vi "FPGA_OffResonanceTapping-SlowScanner.vi"() -> ()   [LabVIEW 2016]
uses:
  <vilib>/rvi/DataTransferAndStorage/Container/XNode/niFpgaContainer.xnode
  <vilib>/rvi/Memory/Memory_Emulation/nirvimemoryEmulation.vi
  <vilib>/rvi/Memory/Memory_Emulation/nirvimemoryFastEmulation.vi
  <vilib>/Platform/TimedLoop/XDataNode/wakeup.ctl
  <vilib>/Platform/TimedLoop/XDataNode/XDNodeRunTimeDep.lvlib
  <vilib>/Platform/TimedLoop/XDataNode/nitl_modes.ctl
  <vilib>/Platform/TimedLoop/XDataNode/timing_clust.ctl
  <vilib>/Platform/TimedLoop/XDataNode/XDataNode.xnode
  <vilib>/eio/EIONode/EIONode.xnode
  <vilib>/rvi/eio/common/nirviEmuTemplateMethod_errors.vi
  <vilib>/rvi/DataTransferAndStorage/Handshake/Emulation/niFpgaHandshakeEmulation.vi
  <vilib>/rvi/FIFO/Fifo_Resource/nirvififoEmulationWrite.vi
  <vilib>/rvi/FIFO/Fifo_Resource/nirvififoEmulationRead.vi
  <vilib>/rvi/FXPMathLib/FxpAdd/XNode/nifxpmath_Add.xnode
  <vilib>/rvi/FXPMathLib/sim/FxpSim.dll
  <instrlib>/_niInstr/Basic Elements/v1/FPGA/niInstr Basic Elements v1 FPGA.lvlib
  <vilib>/rvi/DataTransferAndStorage/Register/Emulation/niFpgaRegisterEmulation.vi
  <vilib>/rvi/interface/RandomDataEmulation/nirviRandomDataFpgaReadWriteTemplate.vi
  <vilib>/rvi/FXPMathLib/FxpInterpret/XNode/nifxpmath_Interpret.xnode
  <vilib>/rvi/FXPMathLib/FxpSub/XNode/nifxpmath_Sub.xnode
  <vilib>/rvi/FXPMathLib/FxpMul/XNode/nifxpmath_Multiplier.xnode
panel:
  out "ticksPerPixel 2":u32
  in  "Tab Control":T1(tab)
  in  "fastBlanking":T2={"startFwd"=0, "endFwd"=10000, "startBwd"=0, "endBwd"=0, "disableBlanking"=FALSE}
  in  "scanRates":T3={"outputRate"=50, "fastDecFactor"=0, "outWaveSizeFast"=0, "pplUpsampling"=0, "numLines"=0}
  in  "scanSize":T4
  in  "outputMatrix":T5
  in  "singleDirectionScan":bool
  in  "scanOffset":cluster{"x":fxp<+/-,16,1>, "y":fxp<+/-,16,1>}
  in  "scanEnabled":bool
  out "actualOutputRate":u32
  in  "fastDecFactorInv":fxp<+,22,0>
  in  "slowUpStep":fxp<+,22,0>
  in  "outWaveSizeSlow":u16
  in  "moveRates":T6
  out "isSlowlyMoving?":bool
  in  "invMoveToDec":fxp<+,16,0>
  in  "moveToPoint":cluster{"x":fxp<+/-,16,1>, "y":fxp<+/-,16,1>}
  in  "doSlowMove":bool
  in  "enableFeedback":bool
  out "zHeightFlt":fxp<+/-,20,2>
  in  "feedbackParams":T7={"setPoint"=0.001007080078125, "pGain"=0.0, "iGain"=0.10000038146972656, "gainScale"=3}
  in  "liftOffParams":T8={"liftHeight"=0.0498046875, "disengagePos"=-1.0}
  out "isPIDatLimit?":bool
  out "inputPID":fxp<+/-,24,1> format="%#_6p"
  out "inputPIDnoRescale":fxp<+/-,24,16>
  in  "manualMotionZ":T9
  out "isManualPIDMoving?":bool
  out "zHeight":fxp<+/-,28,1>
  in  "limits":T10={"upperLimit"=2.0, "lowerLimit"=0.0}
  in  "stepMot.HalfStep":T11={"Address (0-7)"=0, "stateData"=[TRUE, FALSE, FALSE, FALSE], "isWritingToMotor?"=FALSE}
  in  "stepMot.Address(0-7)":i8
  in  "scannerTimeConstant":u32=1000 caption="scanner Time Constant [us]"
  in  "resetBGC":bool
  in  "bgSatCntP2":u16=12
  in  "bgcWaitTicks":u32
  in  "allowPXIBGC":bool
  out "output":cluster{"index":u16, "data":i16}
  out "interactionMaxOut":fxp<+/-,24,16>
  in  "waveLength":u16=5000
  out "readInteraction":i16
  out "readBackground":i16
  in  "readBackgroundAddress":u32
  in  "Count(mSec)":u32=200 caption="updateRateMs"
  in  "intOutMAEnable":bool
  in  "intOutMAExpFactor":i8=-4
  in  "fittingParams":T12={"maxLoc"=0, "threshold"=0, "fitHardPtLimit"=5000}
  in  "outWaveWrite":cluster{"write":bool, "data":i16, "index":u16}
  in  "fitWeightsWrite":T13
  in  "fitFactorWrite":T14
  in  "moveWaveWrite":T15
  in  "moveToWaveWrite":T16
  in  "slowWaveWrite":T17
  in  "fastWaveWrite":T17
  out "X (fast)":i16
  out "Y (slow)":i16
  in  "sosBypass":bool[](array[boolean])=[FALSE, FALSE, FALSE, FALSE, FALSE, FALSE, FALSE, FALSE]
  in  "anot":fxp<+/-,24,5>[](array[numeric])=[0.0, 0.0, 0.0, 0.0, 0.0, 0.0, 0.0, 0.0, 0.0, 0.0, 0.0, 0.0, 0.0, 0.0, 0.0, 0.0]
  in  "b":fxp<+/-,24,5>[](array[numeric])=[0.0, 0.0, 0.0, 0.0, 0.0, 0.0, 0.0, 0.0, 0.0, 0.0, 0.0, 0.0, 0.0, 0.0, 0.0, 0.0, 0.0, 0.0, 0.0, 0.0, 0.0, 0.0, 0.0, 0.0]
  in  "enableOutputSS":bool
  in  "outputSSRate":u16=1000
  out "ticksPerPixel":u32
  out "hostTransferOverflow":bool
  in  "transferInteraction":bool
  in  "syncDecimation":u16=50
  in  "zeroInput":bool
  in  "bypassMaxAveraging":bool
  out "savedPoint":T18
  in  "EnableExcitation":bool
  in  "piezoMode":bool
  in  "invertOutput":bool
  in  "invertInput":bool
  in  "maxSearchBounds":T19={"maxSearchLower"=200, "maxSearchUpper"=600}
  in  "useSyncPoint":bool
  in  "syncPoint":u16
  in  "syncAverageBand":u16=2 caption="syncAverageBand (2^n)"
  out "maxSearchIndex":u16
  in  "zDataRate":u32=45 caption="Count(Ticks)"
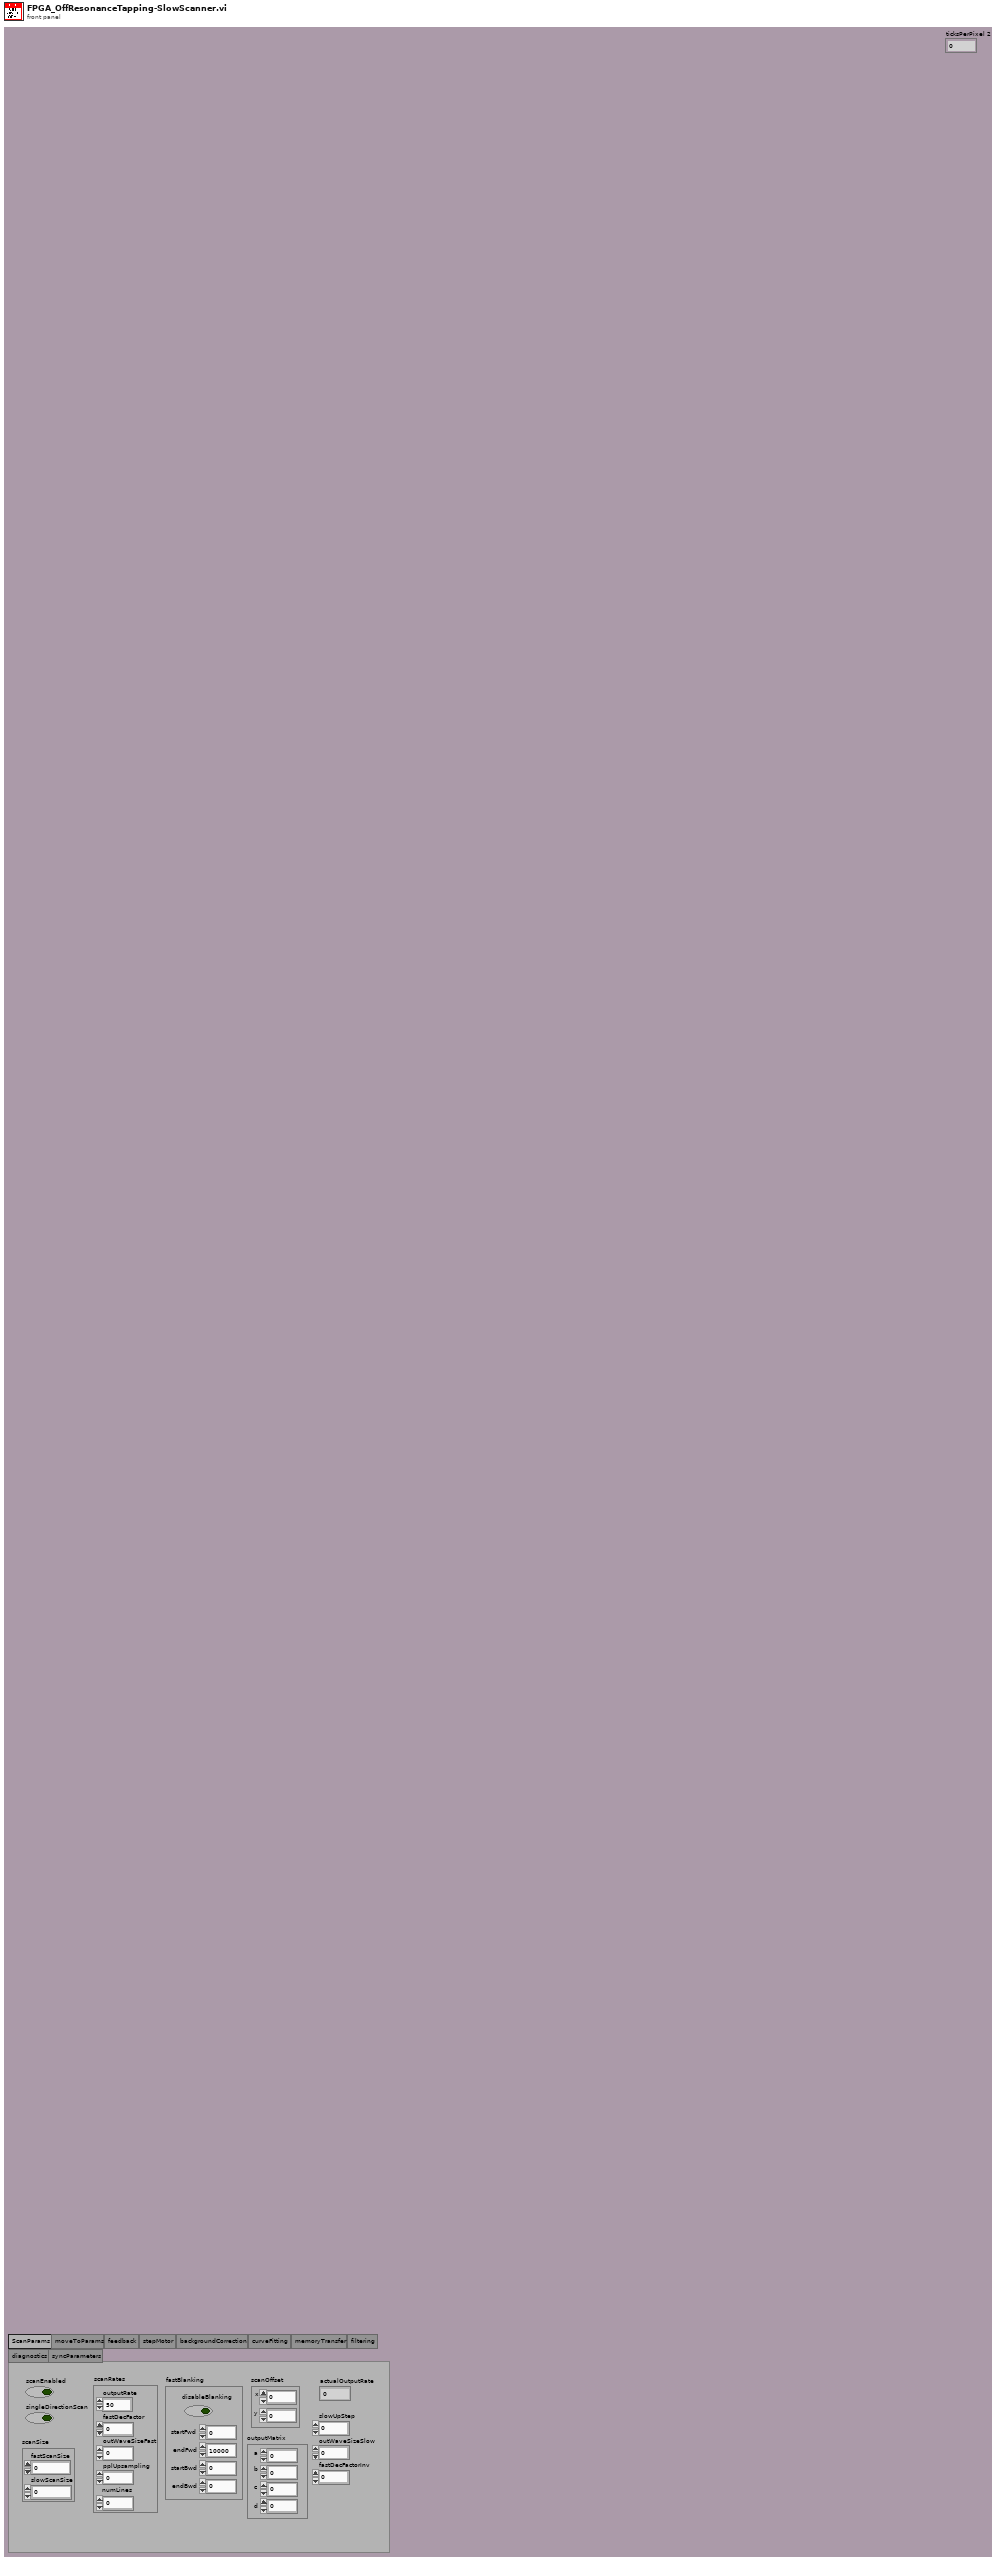
[diagram p1: front panel]
types:
  T1 = enum32{"ScanParams", "moveToParams", "feedback", "stepMotor", "backgroundCorrection", "curveFitting", "memoryTransfer", "filtering", "diagnostics", "syncParameters"}
  T2 = cluster{"startFwd":u16, "endFwd":u16, "startBwd":u16, "endBwd":u16, "disableBlanking":bool}
  T3 = cluster{"outputRate":u16, "fastDecFactor":u16, "outWaveSizeFast":u16, "pplUpsampling":u16, "numLines":u16}
  T4 = cluster{"fastScanSize":fxp<+,17,1>, "slowScanSize":fxp<+,17,1>}
  T5 = cluster{"a":fxp<+/-,18,2>, "b":fxp<+/-,18,2>, "c":fxp<+/-,18,2>, "d":fxp<+/-,18,2>}
  T6 = cluster{"moveToDecFactor":u16, "moveToWaveSize":u16}
  T7 = cluster{"setPoint":fxp<+/-,17,1>, "pGain":fxp<+/-,20,1>, "iGain":fxp<+/-,20,1>, "gainScale":i8}
  T8 = cluster{"liftHeight":fxp<+/-,15,4>, "disengagePos":fxp<+/-,22,1>}
  T9 = cluster{"enableManualMotion":bool, "doMove":bool, "integratorTarget":fxp<+/-,22,2>, "moveDecimation":u16, "moveWaveSize":u16}
  T10 = cluster{"upperLimit":fxp<+/-,28,4>, "lowerLimit":fxp<+/-,28,4>}
  T11 = cluster{"Address (0-7)":u8, "stateData":bool[], "isWritingToMotor?":bool}
  T12 = cluster{"maxLoc":u16, "threshold":i16, "fitHardPtLimit":u16}
  T13 = cluster{"write":bool, "data":fxp<+,20,0>, "index":u16}
  T14 = cluster{"write":bool, "index":u16, "fitCoefficients":cluster{"a":fxp<+/-,21,7>, "b":fxp<+/-,21,7>, "factorA":i8, "factorB":i8}}
  T15 = cluster{"write":bool, "data":fxp<+,16,1>, "index":u16}
  T16 = cluster{"write":bool, "index":u16, "data":fxp<+/-,18,1>}
  T17 = cluster{"write":bool, "index":u16, "data":fxp<+/-,18,2>}
  T18 = cluster{"xOut":fxp<+/-,18,2>, "yOut":fxp<+/-,18,2>}
  T19 = cluster{"maxSearchLower":u16, "maxSearchUpper":u16}
  T20 = typedef "XDNodeRunTimeDep.lvlib/timing_clust.ctl" = cluster{"Expected End [f-1]":u64, "Actual End [f-1]":u64, "Finished Late? [f-1]":bool, "Expected End [i-1]":u64, "Actual End [i-1]":u64, "Finished Late? [i-1]":bool, "Expected Start [i]":u64, "Actual Start [i]":u64, "Expected Start [f]":u64, "Actual Start [f]":u64, "Source Name":string, "Structure Name":string, "Period":i64, "Deadline":i64, "Offset":i64, "Start":i64, "Priority":i32, "Timeout":i32, "Mode":T21, "Wakeup Reason":T22, "Error":errorcluster, "Source Type":string, "Secondary Source Type":string, "Global End Time":u64, "Global Start Time":u64, "Frame Duration":u64, "Iteration Duration":u64, "Assigned CPU":i32, "I/O Scan Engine Mode":u32}
  T21 = typedef "XDNodeRunTimeDep.lvlib/nitl_modes.ctl" = enum32{"No Change", "Process missed periods, maintain original phase", "Discard missed periods, maintain original phase", "Process missed periods, ignore original phase", "Discard missed periods, ignore original phase"}
  T22 = typedef "XDNodeRunTimeDep.lvlib/wakeup.ctl" = enum32{"Normal", "Aborted", "Asynchronous wakeup", "Timing source error", "Timed loop error", "Timeout"}
  T23 = cluster{"linSum":i32, "wtSum":fxp<+/-,54,34>, "count":u16, "forward":bool}
  T24 = cluster{cluster{"outMinFwd":fxp<+,22,1>, "outMinBwd":fxp<+,22,1>}, "outputValid":bool}
  T25 = cluster{"Element":cluster{"a":i32, "b":i32}, "outputValid":bool}
  T26 = cluster{"Element":cluster{"linSum":i32, "wtSum":fxp<+/-,54,34>, "count":u16}, "outputValid":bool}
  T27 = cluster{"outMinFwd":fxp<+,22,1>, "outMinBwd":fxp<+,22,1>}
  T28 = cluster{"linSum":i32, "wtSum":fxp<+/-,54,34>, "count":u16}
  T29 = cluster{"enable":bool, "setPoint":fxp<+/-,17,1>, "pGain":fxp<+/-,20,1>, "iGain":fxp<+/-,20,1>, "gainScale":i8}
  T30 = cluster{"liftHeight":fxp<+/-,15,4>, "disengagePos":fxp<+/-,22,1>, "liftOff":bool}
  T31 = cluster{"zHeight":fxp<+/-,28,1>, "integer_zHeight":i16, "error":fxp<+/-,25,2>, "pidAtLimit":bool, "moving":bool}
  T32 = cluster{"a":fxp<+/-,21,7>, "b":fxp<+/-,21,7>, "factorA":i8, "factorB":i8}
  T33 = cluster{"output":bool, "fastIndex":bool, "line":bool, "frame":bool, "moveIndex":bool, "moveDone":bool, "pixel":bool}
  T34 = cluster{"interpOutput":fxp<+/-,19,2>, "interpOutput":fxp<+/-,19,2>}
  T35 = cluster{"x+y":fxp<+/-,18,2>, "x+y":fxp<+/-,18,2>}
  T36 = cluster{"[0]":bool, "[1]":bool, "[2]":bool, "[3]":bool, "[4]":bool, "[5]":bool, "[6]":bool, "[7]":bool, "[8]":bool}
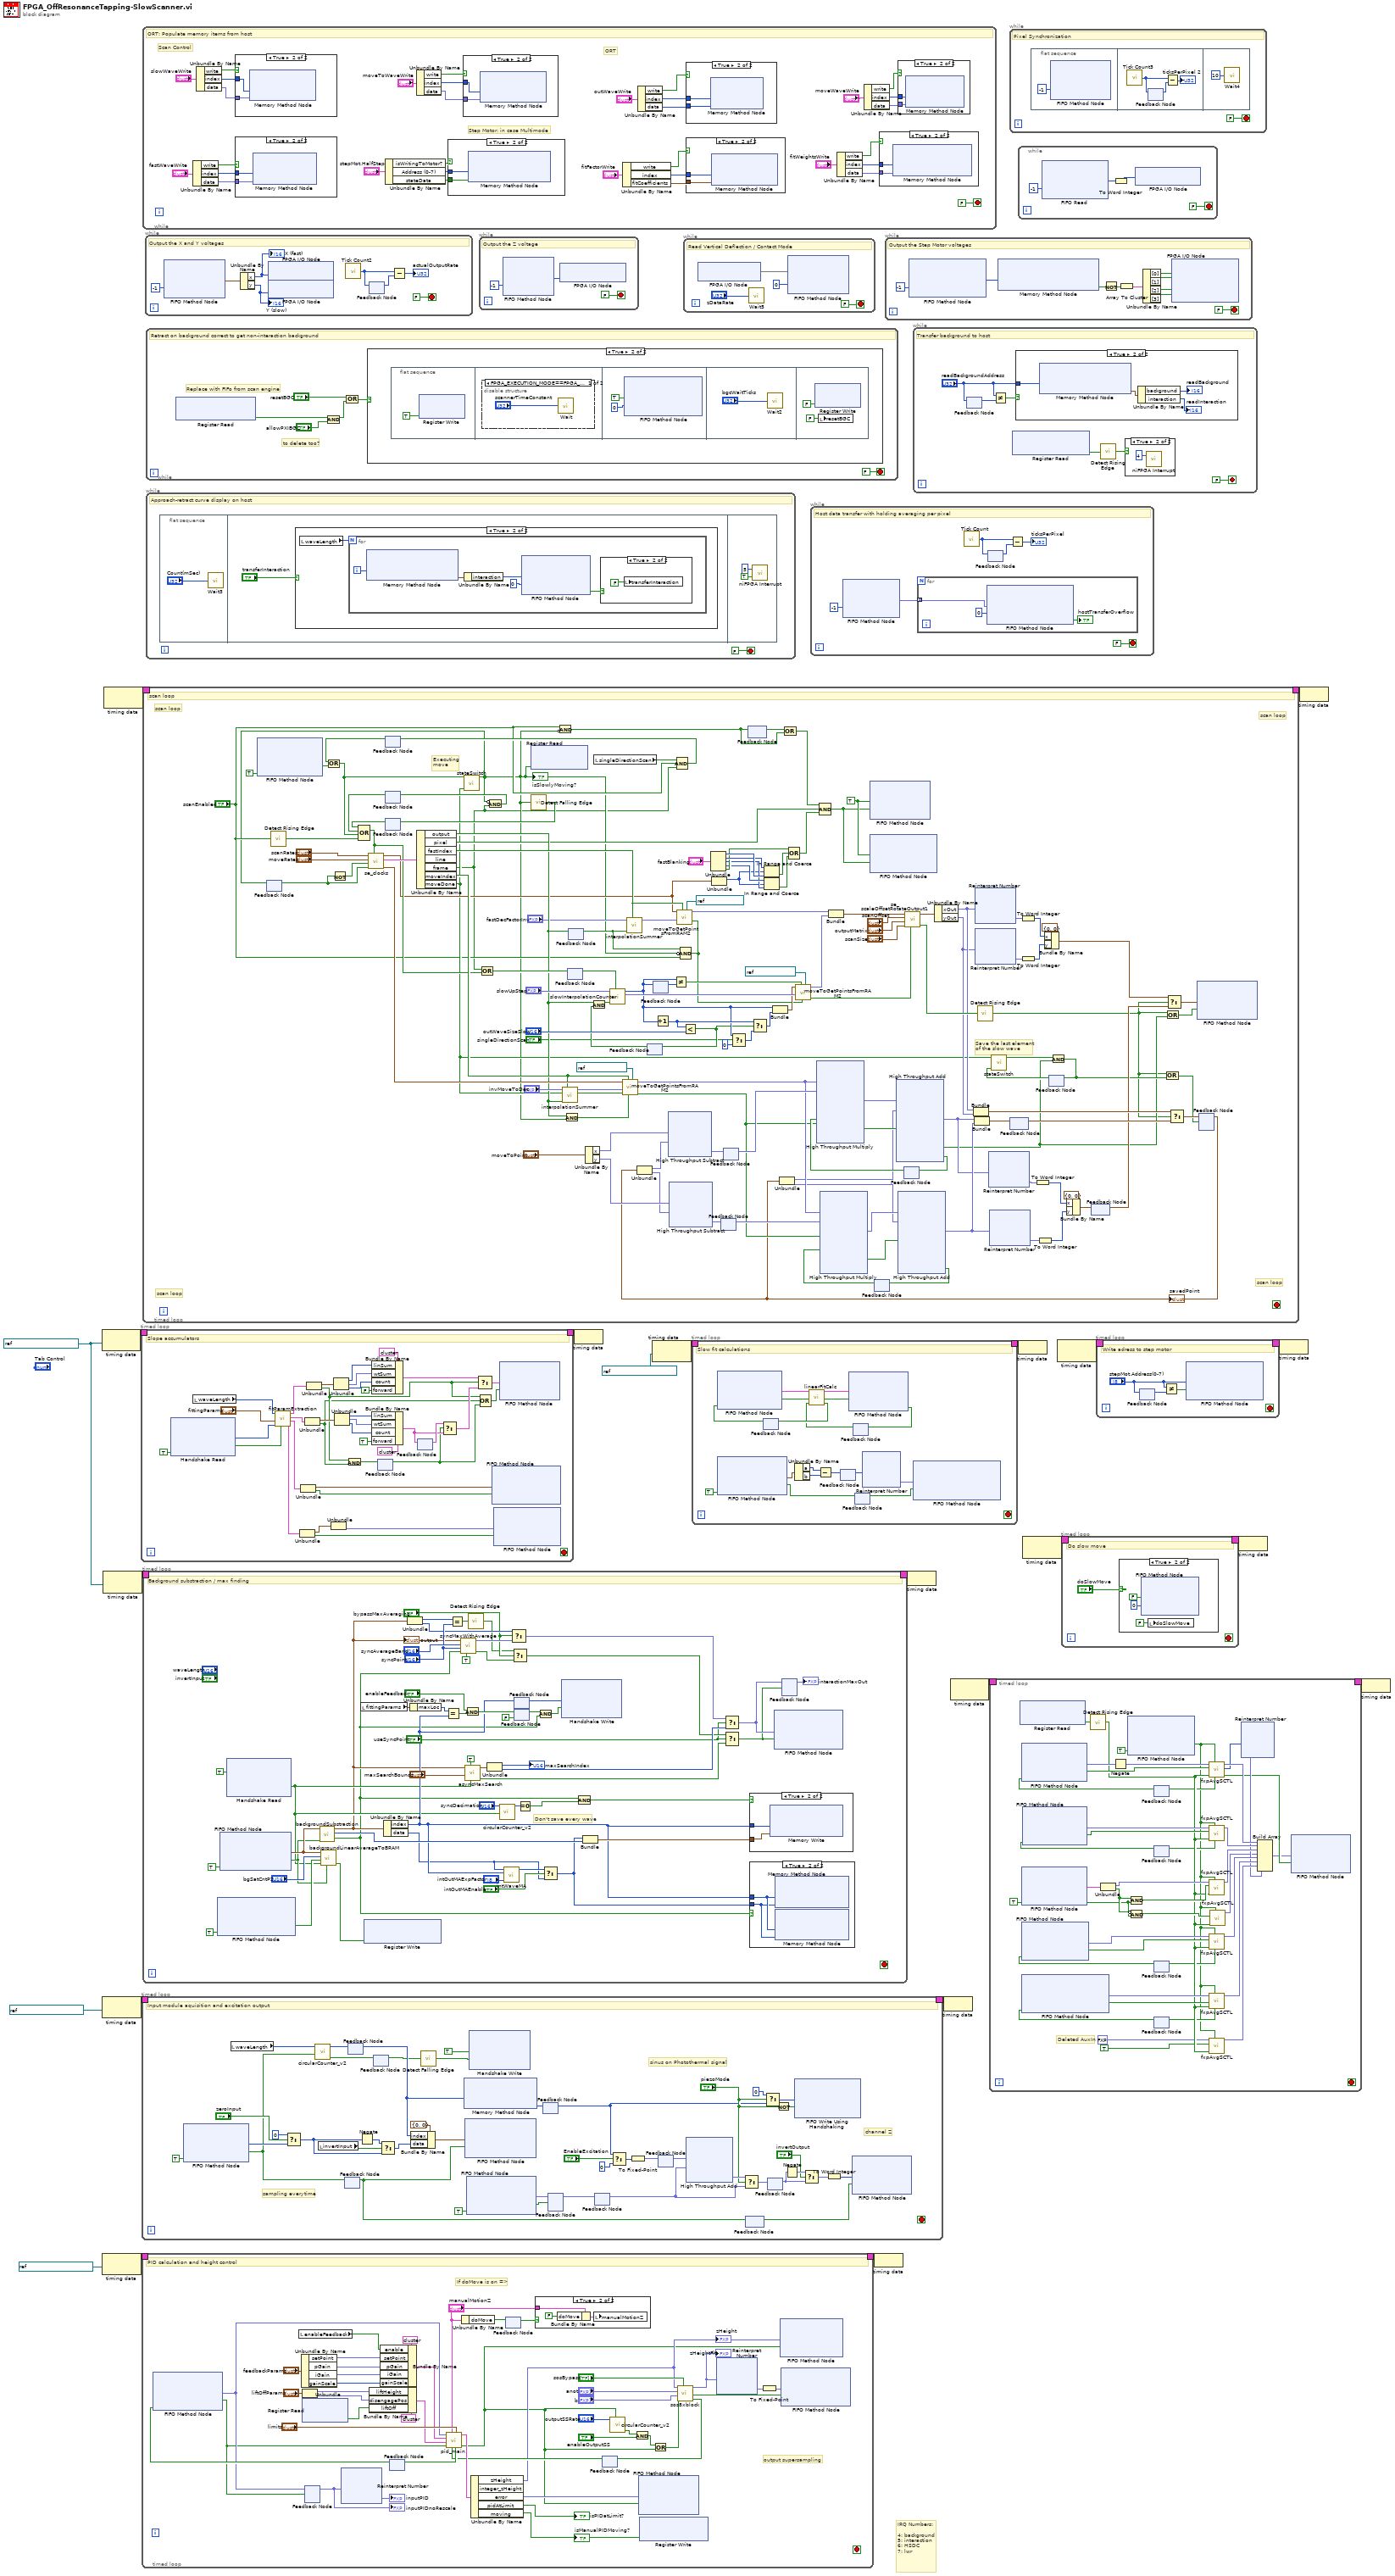
[diagram p0: block diagram]
diagram:
  w7 = refnum<k21> "40 MHz Onboard Clock" ("Source Name")
  # "IRQ Numbers:\n\n4: background\n5: interaction\n6: HSDC\n7: lwr"
  n1 = node-c288(w7) -> (w18:T20)
  n2 = node-c288(refnum<k21> "40 MHz Onboard Clock" ("Source Name")) -> (w22:T20)
  n3 = node-c288(refnum<k21> "40 MHz Onboard Clock" ("Source Name")) -> (w16:T20)
  n4 = node-c288(w7) -> (w20:T20)
  n5 = node-c288() -> (w4:T20)  [unwired: 1 in]
  n6 = timed-loop {
    timing: w18 -> [_]
    timing-out: [_] -> w17
    stop <- _ stop-if-true
    # "Slope accumulators"
    n7 = xnode ("Handshake Read")("Ready for Output"=TRUE) -> ("Data"=w57:u16, "Output Valid"=w56:bool)  [unwired: 1 in, 1 out]
    n8 = local read "waveLength"() -> (w54:u16)
    n9 = call "fitParamExtraction.vi"("startFit"=w56, "startIndex"=w57, "fittingParams"="fittingParams", "waveLength"=w54) -> ("minValues"=w26:T24, "integralParts"=w29:T25, "fitFwd"=w45:T26, "fitBwd"=w52:T26)  [unwired: 4 in]
    n10 = Unbundle(w26) -> (w25:T27, "outputValid"=w23:bool)
    n11 = Unbundle(w29) -> ("Element"=w28:cluster{"a":i32, "b":i32}, "outputValid"=w27:bool)
    n12 = Unbundle(w45) -> ("Element"=w44:T28, "outputValid"=w31:bool)
    n13 = Unbundle(w52) -> ("Element"=w51:T28, "outputValid"=w32:bool)
    n14 = Unbundle(w25) -> ("outMinBwd"=w24:fxp<+,22,1>)  [unwired: 1 out]
    n15 = Unbundle(w51) -> ("linSum"=w50:i32, "wtSum"=w49:fxp<+/-,54,34>, "count"=w48:u16)
    n16 = Unbundle(w44) -> ("linSum"=w41:i32, "wtSum"=w40:fxp<+/-,54,34>, "count"=w39:u16)
    n17 = And(x=w32, y=w31) -> (x .and. y?=w37:bool)
    n18 = Bundle By Name(cluster=T23 {"linSum"=0, "wtSum"=0.0, "count"=0, "forward"=FALSE} ("Element"), "linSum"=w50, "wtSum"=w49, "count"=w48, "forward"=FALSE) -> (w46:T23)
    n19 = Bundle By Name(cluster=T23 {"linSum"=0, "wtSum"=0.0, "count"=0, "forward"=FALSE} ("Element"), "linSum"=w41, "wtSum"=w40, "count"=w39, "forward"=TRUE) -> (w34:T23)
    n20 = feedback #1() -> (w30:bool)  [unwired: 1 in]
    n21 = feedback-in #1(w37) -> ()
    n22 = feedback-in #2(w34) -> ()
    n23 = feedback #2() -> (w35:T23)  [unwired: 1 in]
    n24 = Select(t=w35, s=w30, f=w34) -> (s? t:f=w36:T23)
    n25 = Select(t=w46, s=w32, f=w36) -> (s? t:f=w38:T23)
    n26 = Compound Arithmetic op=OR(w32, w31, w30) -> (w33:bool)
    n27 = xnode ("FIFO Method Node")("Element"=w28, "Input Valid"=w27) -> ()  [unwired: 1 in, 2 out]
    n28 = xnode ("FIFO Method Node")("Element"=w24, "Input Valid"=w23) -> ()  [unwired: 1 in, 2 out]
    n29 = xnode ("FIFO Method Node")("Element"=w38, "Input Valid"=w33) -> ()  [unwired: 1 in, 2 out]
  }
  n30 = timed-loop {
    timing: w22 -> [_]
    timing-out: [_] -> w21
    stop <- _ stop-if-true
    # "sampling everytime"
    # "sinus on Photothermal signal"
    # "channel Z"
    # "Input module aquisition and excitation output"
    n31 = xnode ("FIFO Method Node")("Ready for Output"=TRUE) -> ("Element"=w74:i16, "Output Valid"=w71:bool)  [unwired: 1 in, 1 out]
    n32 = local read "waveLength"() -> (w96:u16)
    n33 = Select(t=i16 0, s="zeroInput", f=w74) -> (s? t:f=w77:i16)
    n34 = call "circularCounter_v2.vi"("doStep"=w71, "maxCount"=w96) -> ("maxReached"=w95:bool, "index"=w84:u16)  [unwired: 6 in, 2 out]
    n35 = local read "invertInput"() -> (w97:bool)
    n36 = feedback-in #3(w71) -> ()
    n37 = feedback #3() -> (w69:bool)  [unwired: 1 in]
    n38 = feedback-in #4(w84) -> ()
    n39 = feedback #4() -> (w87:u16)  [unwired: 1 in]
    n40 = Negate(x=w77) -> (-x=w98:i16)
    n41 = feedback-in #5(w95) -> ()
    n42 = feedback #5() -> (w86:bool)  [unwired: 1 in]
    n43 = Select(t=w98, s=w97, f=w77) -> (s? t:f=w99:i16)
    n44 = Bundle By Name(cluster=cluster{"index":u16, "data":i16} {"index"=0, "data"=0} ("dataPair"), "index"=w87, "data"=w99) -> (w100:cluster{"index":u16, "data":i16})
    n45 = call <instrlib>:"Detect Falling Edge.vi"("signal"=w86) -> ("edge detected"=w85:bool)  [unwired: 14 in]
    n46 = xnode ("Memory Method Node")("Address"=w87) -> ("Data"=w101:i16)  [unwired: 1 in, 1 out]
    n47 = xnode ("FIFO Method Node")("Element"=w100, "Input Valid"=w69) -> ()  [unwired: 1 in, 2 out]
    n48 = xnode ("FIFO Method Node")("Ready for Output"=TRUE) -> ("Element"=w93:fxp<+/-,18,16>, "Output Valid"=w94:bool)  [unwired: 1 in, 1 out]
    n49 = xnode ("Handshake Write")("Data"=TRUE, "Input Valid"=w85) -> ()  [unwired: 1 in, 2 out]
    n50 = feedback #6() -> (w62:i16)  [unwired: 1 in]
    n51 = feedback-in #6(w101) -> ()
    n52 = feedback-in #7(w93, w94) -> ()
    n53 = feedback #7() -> (w78:fxp<+/-,18,16>)  [unwired: 1 in]
    n54 = feedback-in #8(w78) -> ()
    n55 = feedback #8() -> (w76:fxp<+/-,18,16>)  [unwired: 1 in]
    n56 = Select(t=w62, s="EnableExcitation", f=i16 0 ("t")) -> (s? t:f=w66:i16)
    n57 = To Fixed-Point(number=w66) -> (fixed-point=w90:fxp<+/-,16,16>)  [unwired: 1 in]
    n58 = feedback-in #9(w90) -> ()
    n59 = feedback #9() -> (w88:fxp<+/-,16,16>)  [unwired: 1 in]
    n60 = xnode ("High Throughput Add")("x"=w88, "y"=w76) -> ("x+y"=w89:fxp<+/-,18,16>)
    n61 = Select(t=w89, s="piezoMode", f=w76) -> (s? t:f=w91:fxp<+/-,18,16>)
    n62 = feedback-in #10(w69) -> ()
    n63 = feedback #10() -> (w68:bool)  [unwired: 1 in]
    n64 = Select(t=i16 0, s="piezoMode", f=w62) -> (s? t:f=w72:i16)
    n65 = feedback-in #11(w91) -> ()
    n66 = feedback #11() -> (w81:fxp<+/-,18,16>)  [unwired: 1 in]
    n67 = Not(x="piezoMode") -> (.not. x?=w64:bool)
    n68 = Negate(x=w81) -> (-x=w80:fxp<+/-,19,17>)
    n69 = xnode ("FIFO Write Using Handshaking")("Element"=w72, "Input Valid"=w64) -> ()  [unwired: 1 in, 2 out]
    n70 = Select(t=w80, s="invertOutput", f=w81) -> (s? t:f=w70:fxp<+/-,19,17>)
    n71 = To Word Integer(number=w70) -> (16bit integer=w67:i16)
    n72 = xnode ("FIFO Method Node")("Element"=w67, "Input Valid"=w68) -> ()  [unwired: 1 in, 2 out]
  }
  n73 = timed-loop {
    timing: w16 -> [_]
    timing-out: [_] -> w15
    stop <- _ stop-if-true
    # "If doMove is on =>"
    # "output supersampling"
    # "PID calculation and height control"
    n74 = local read "enableFeedback"() -> (w116:bool)
    n75 = Unbundle By Name("feedbackParams") -> ("setPoint"=w106:fxp<+/-,17,1>, "pGain"=w130:fxp<+/-,20,1>, "iGain"=w129:fxp<+/-,20,1>, "gainScale"=w128:i8)
    n76 = Unbundle("liftOffParams") -> ("liftHeight"=w141:fxp<+/-,15,4>, "disengagePos"=w140:fxp<+/-,22,1>)
    n77 = xnode ("Register Read")() -> ("Data"=w139:bool)  [unwired: 1 in, 1 out]
    n78 = feedback #12() -> (w133:fxp<+/-,24,16>)  [unwired: 1 in]
    "inputPIDnoRescale" <- w133
    n79 = xnode "Reinterpret Number"("x"=w133) -> ("y"=→"inputPID":fxp<+/-,24,1>)
    n80 = Bundle By Name(cluster=T30 {"liftHeight"=0.0498046875, "disengagePos"=-1.0, "liftOff"=FALSE} ("liftOffParams"), "liftHeight"=w141, "disengagePos"=w140, "liftOff"=w139) -> (w138:T30)
    n81 = Bundle By Name(cluster=T29 {"enable"=FALSE, "setPoint"=0.001007080078125, "pGain"=0.0, "iGain"=0.10000038146972656, "gainScale"=0} ("fbParams"), "enable"=w116, "setPoint"=w106, "pGain"=w130, "iGain"=w129, "gainScale"=w128) -> (w115:T29)
    n82 = feedback #13() -> (w148:bool)  [unwired: 1 in]
    n83 = xnode ("FIFO Method Node")("Ready for Output"=w148) -> ("Element"=w135:fxp<+/-,24,16>, "Output Valid"=w110:bool)  [unwired: 1 in, 1 out]
    n84 = feedback-in #12(w135, w110) -> ()
    n85 = Unbundle By Name("manualMotionZ") -> ("doMove"=w112:bool)
    n86 = feedback-in #14(w112) -> ()
    n87 = feedback #14() -> (w109:bool)  [unwired: 1 in]
    n88 = case shown="True" w109 {
      tunnel: "manualMotionZ" -> [_ w152]
      frame False {
      }
      frame True {
        n89 = Bundle By Name(cluster=w152, "doMove"=FALSE) -> (w150:T9)
        n90 = local write "manualMotionZ"(w150) -> ()
      }
    }
    n91 = feedback #15() -> (w145:bool)  [unwired: 1 in]
    n92 = call "pid_main.vi"("Z.Voltagelimits (0-2)"="limits", "ready for output (T)"=w145, "manualMotionZ"="manualMotionZ", "input valid"=w110, "liftOffParams"=w138, "fbParams"=w115, "input"=w135) -> ("output valid"=w107:bool, "output"=w146:T31, "ready for input"=w147:bool)  [unwired: 2 in]
    n93 = feedback-in #13(w147) -> ()
    n94 = Unbundle By Name(w146) -> ("zHeight"=w108:fxp<+/-,28,1>, "error"=w144:fxp<+/-,25,2>, "pidAtLimit"=→"isPIDatLimit?":bool, "moving"=w111:bool)  [unwired: 1 out]
    "isManualPIDMoving?" <- w111
    "zHeight" <- w108
    n95 = call "circularCounter_v2.vi"("reset"=w107, "maxCount"="outputSSRate") -> ("maxReached"=w121:bool)  [unwired: 6 in, 3 out]
    n96 = And(x=w121, y="enableOutputSS") -> (x .and. y?=w118:bool)
    n97 = xnode ("FIFO Method Node")("Element"=w144, "Input Valid"=w107) -> ()  [unwired: 1 in, 2 out]
    n98 = xnode ("Register Write")("Data"=w111) -> ()  [unwired: 1 in, 1 out]
    n99 = Or(x=w118, y=w107) -> (x .or. y?=w119:bool)
    n100 = call "sos8xblock.vi"("sosBypass"="sosBypass", "input valid"=w119, "b"="b", "anot"="anot", "input"=w108) -> ("ready for input"=w124:bool, "output valid"=w123:bool, "output"=w132:fxp<+/-,20,2>)  [unwired: 4 in]
    "zHeightFlt" <- w132
    n101 = feedback-in #15(w124) -> ()
    n102 = xnode "Reinterpret Number"("x"=w132) -> ("y"=w137:fxp<+/-,20,17>)
    n103 = To Fixed-Point(number=w137) -> (fixed-point=w136:fxp<+/-,18,16>)  [unwired: 1 in]
    n104 = xnode ("FIFO Method Node")("Element"=w108, "Input Valid"=w107) -> ()  [unwired: 1 in, 2 out]
    n105 = xnode ("FIFO Method Node")("Element"=w136, "Input Valid"=w123) -> ()  [unwired: 1 in, 2 out]
  }
  n106 = timed-loop {
    timing: w20 -> [_]
    timing-out: [_] -> w19
    stop <- _ stop-if-true
    # "Don't save every wave"
    # "Background substraction / max finding"
    n107 = xnode ("FIFO Method Node")("Ready for Output"=TRUE) -> ("Output Valid"=w190:bool)  [unwired: 1 in, 2 out]
    n108 = xnode ("FIFO Method Node")("Ready for Output"=TRUE) -> ("Element"=w208:cluster{"index":u16, "data":i16}, "Output Valid"=w162:bool)  [unwired: 1 in, 1 out]
    n109 = xnode ("Handshake Read")("Ready for Output"=TRUE) -> ("Output Valid"=w157:bool)  [unwired: 1 in, 2 out]
    n110 = call "backgroundSubstraction.vi"("inputValid"=w162, "input"=w208) -> ("outptValid"=w155:bool, "background"=w189:i16, "output"=w156:cluster{"index":u16, "data":i16})  [unwired: 7 in]
    "output" <- w156
    n111 = call "backgroundLinearAverageToBRAM.vi"("inputValid"=w162, "endOfWave"=w157, "startRecording"=w190, "bgSatCntP2"="bgSatCntP2", "input"=w208) -> ("backgroundReady"=w191:bool)  [unwired: 5 in, 1 out]
    n112 = local read "fittingParams"() -> (w203:T12)
    n113 = xnode ("Register Write")("Data"=w191) -> ()  [unwired: 1 in, 1 out]
    n114 = Unbundle By Name(w156) -> ("index"=w159:u16, "data"=w158:i16)
    n115 = Unbundle(w156) -> ("index"=w181:u16, "data"=w179:i16)
    n116 = Unbundle By Name(w203) -> ("maxLoc"=w202:u16)
    n117 = Equal?(x=w202, y=w159) -> (x = y?=w160:bool)
    n118 = Equal?(x=w181, y="syncPoint") -> (x = y?=w180:bool)
    n119 = call "syncMaxWithAverage.vi"("enable"=TRUE, "inputValid"=w155, "syncPoint"="syncPoint", "syncAverageBand"="syncAverageBand", "input"=w156) -> ("outputValid"=w183:bool, "waveMaxAvg"=w196:fxp<+/-,24,16>)  [unwired: 5 in]
    n120 = call "asyncMaxSearch.vi"("reset"=w157, "enable"=TRUE, "maxSearchBounds"="maxSearchBounds", "inputPair"=w156) -> ("outputValid"=w176:bool, "output"=w195:cluster{"index":u16, "data":i16})  [unwired: 6 in]
    n121 = And(x="enableFeedback", y=w160) -> (x .and. y?=w198:bool)
    n122 = call <instrlib>:"Detect Rising Edge.vi"("signal"=w180) -> ("edge detected"=w177:bool)  [unwired: 14 in]
    n123 = Unbundle(w195) -> ("index"=→"maxSearchIndex":u16, "data"=w175:i16)
    n124 = call "circularCounter_v2.vi"("doStep"=w157, "maxCount"="syncDecimation") -> ("index"=w204:u16)  [unwired: 6 in, 3 out]
    n125 = call "intWaveMA.vi"("expFactor"="intOutMAExpFactor", "Address"=w159, "update"=w158) -> ("output"=w166:i16)  [unwired: 8 in]
    n126 = Select(t=w179, s="bypassMaxAveraging", f=w196) -> (s? t:f=w173:fxp<+/-,24,16>)
    n127 = Select(t=w177, s="bypassMaxAveraging", f=w183) -> (s? t:f=w174:bool)
    n128 = feedback #16() -> (w200:u16)  [unwired: 1 in]
    n129 = feedback-in #16(w159) -> ()
    n130 = feedback #17(FALSE) -> (w201:bool)
    n131 = feedback-in #17(w198) -> ()
    n132 = Equal To 0?(x=w204) -> (x = 0?=w206:bool)
    n133 = Compound Arithmetic op=AND(w201, w155) -> (w186:bool)
    n134 = Select(t=w166, s="intOutMAEnable", f=w158) -> (s? t:f=w163:i16)
    n135 = xnode ("Handshake Write")("Data"=w200, "Input Valid"=w186) -> ()  [unwired: 1 in, 2 out]
    n136 = Compound Arithmetic op=AND(w155, w206) -> (w187:bool)
    n137 = Bundle("data"=w163, "background"=w189) -> (w188:cluster{"data":i16, "background":i16})  [unwired: 1 in]
    n138 = Select(t=w173, s="useSyncPoint", f=w175) -> (s? t:f=w168:fxp<+/-,24,16>)
    n139 = Select(t=w174, s="useSyncPoint", f=w176) -> (s? t:f=w167:bool)
    n140 = case shown="True" w187 {
      tunnel: w159 -> [_ w212]
      tunnel: w188 -> [_ w211]
      frame False {
      }
      frame True {
        n141 = xnode ("Memory Write")("Address"=w212, "Data"=w211) -> ()  [unwired: 1 in, 1 out]
      }
    }
    n142 = case shown="True" w155 {
      tunnel: w159 -> [_ w210]
      tunnel: w163 -> [_ w209]
      frame False {
      }
      frame True {
        n143 = xnode ("Memory Method Node")("Address"=w210, "Data"=w209) -> ()  [unwired: 1 in, 1 out]
        n144 = xnode ("Memory Method Node")("Address"=w210, "Data"=w209) -> ()  [unwired: 1 in, 1 out]
      }
    }
    n145 = xnode ("FIFO Method Node")("Element"=w168, "Input Valid"=w167) -> ()  [unwired: 1 in, 2 out]
    n146 = feedback #18() -> (→"interactionMaxOut":fxp<+/-,24,16>)  [unwired: 1 in]
    n147 = feedback-in #18(w168, w167) -> ()
  }
  n148 = while {
    stop <- FALSE stop-if-true
    # "Scan Control"
    # "ORT"
    # "Step Motor: in case Multimode"
    # "ORT: Populate memory items from host"
    n149 = Unbundle By Name("fastWaveWrite") -> ("write"=w241:bool, "index"=w240:u16, "data"=w239:fxp<+/-,18,2>)
    n150 = Unbundle By Name("slowWaveWrite") -> ("write"=w243:bool, "index"=w245:u16, "data"=w244:fxp<+/-,18,2>)
    n151 = case shown="True" w241 {
      tunnel: w240 -> [_ w261]
      tunnel: w239 -> [_ w260]
      frame False {
      }
      frame True {
        n152 = xnode ("Memory Method Node")("Address"=w261, "Data"=w260) -> ()  [unwired: 1 in, 1 out]
      }
    }
    n153 = case shown="True" w243 {
      tunnel: w245 -> [_ w263]
      tunnel: w244 -> [_ w262]
      frame False {
      }
      frame True {
        n154 = xnode ("Memory Method Node")("Address"=w263, "Data"=w262) -> ()  [unwired: 1 in, 1 out]
      }
    }
    n155 = Unbundle By Name("stepMot.HalfStep") -> ("isWritingToMotor?"=w231:bool, "Address (0-7)"=w232:u8, "stateData"=w233:bool[])
    n156 = Unbundle By Name("moveToWaveWrite") -> ("write"=w237:bool, "index"=w235:u16, "data"=w236:fxp<+/-,18,1>)
    n157 = case shown="True" w231 {
      tunnel: w233 -> [_ w257]
      tunnel: w232 -> [_ w256]
      frame False {
      }
      frame True {
        n158 = xnode ("Memory Method Node")("Address"=w256, "Data"=w257) -> ()  [unwired: 1 in, 1 out]
      }
    }
    n159 = case shown="True" w237 {
      tunnel: w236 -> [_ w259]
      tunnel: w235 -> [_ w258]
      frame False {
      }
      frame True {
        n160 = xnode ("Memory Method Node")("Address"=w258, "Data"=w259) -> ()  [unwired: 1 in, 1 out]
      }
    }
    n161 = Unbundle By Name("fitFactorWrite") -> ("write"=w223:bool, "index"=w224:u16, "fitCoefficients"=w226:T32)
    n162 = Unbundle By Name("outWaveWrite") -> ("write"=w228:bool, "index"=w229:u16, "data"=w230:i16)
    n163 = case shown="True" w228 {
      tunnel: w229 -> [_ w255]
      tunnel: w230 -> [_ w254]
      frame False {
      }
      frame True {
        n164 = xnode ("Memory Method Node")("Address"=w255, "Data"=w254) -> ()  [unwired: 1 in, 1 out]
      }
    }
    n165 = case shown="True" w223 {
      tunnel: w224 -> [_ w253]
      tunnel: w226 -> [_ w252]
      frame False {
      }
      frame True {
        n166 = xnode ("Memory Method Node")("Address"=w253, "Data"=w252) -> ()  [unwired: 1 in, 1 out]
      }
    }
    n167 = Unbundle By Name("fitWeightsWrite") -> ("write"=w221:bool, "index"=w220:u16, "data"=w219:fxp<+,20,0>)
    n168 = Unbundle By Name("moveWaveWrite") -> ("write"=w216:bool, "index"=w217:u16, "data"=w218:fxp<+,16,1>)
    n169 = case shown="True" w221 {
      tunnel: w220 -> [_ w251]
      tunnel: w219 -> [_ w250]
      frame False {
      }
      frame True {
        n170 = xnode ("Memory Method Node")("Address"=w251, "Data"=w250) -> ()  [unwired: 1 in, 1 out]
      }
    }
    n171 = case shown="True" w216 {
      tunnel: w217 -> [_ w249]
      tunnel: w218 -> [_ w248]
      frame False {
      }
      frame True {
        n172 = xnode ("Memory Method Node")("Address"=w249, "Data"=w248) -> ()  [unwired: 1 in, 1 out]
      }
    }
  }
  n173 = timed-loop {
    timing: w4 -> [_]
    timing-out: [_] -> w3
    stop <- _ stop-if-true
    w350 = TRUE ("Element")
    # "scan loop"
    # "scan loop"
    # "scan loop"
    # "scan loop"
    # "Save the last element \nof the slow wave"
    # "Executing\nmove"
    # "scan loop"
    n174 = xnode ("FIFO Method Node")("Ready for Output"=TRUE) -> ("Output Valid"=w273:bool)  [unwired: 1 in, 2 out]
    n175 = feedback #19() -> (w296:bool)  [unwired: 1 in]
    n176 = call <instrlib>:"Detect Rising Edge.vi"("signal"="scanEnabled") -> ("edge detected"=w271:bool)  [unwired: 14 in]
    n177 = Not(x=w296) -> (.not. x?=w295:bool)
    n178 = feedback #20() -> (w306:bool)  [unwired: 1 in]
    n179 = Compound Arithmetic op=OR(w306, w273) -> (w302:bool)
    n180 = feedback #21() -> (w335:bool)  [unwired: 1 in]
    n181 = feedback #22() -> (w334:bool)  [unwired: 1 in]
    n182 = Compound Arithmetic op=OR(w334, w335, w302, w271) -> (w304:bool)
    n183 = call "se_clocks.vi"("resetClocks"=w304, "stepSlow"=w296, "stepScan"=w295, "moveRates"="moveRates", "scanRates"="scanRates") -> ("moveIndices"=w343:cluster{"index":u16, "next":u16}, "clocks"=w345:T33, "fastIndices"=w285:cluster{"index":u16, "next":u16})  [unwired: 3 in, 1 out]
    n184 = Unbundle By Name(w345) -> ("output"=w290:bool, "pixel"=w288:bool, "fastIndex"=w342:bool, "frame"=w264:bool, "moveIndex"=w341:bool, "moveDone"=w272:bool)  [unwired: 1 out]
    n185 = call "stateSwitch.vi"("disable"=w272, "enable"=w302) -> ("state"=w265:bool)  [unwired: 9 in]
    "isSlowlyMoving?" <- w265
    n186 = feedback-in #19(w265) -> ()
    n187 = Compound Arithmetic op=OR(w264, w304) -> (w305:bool)
    n188 = Compound Arithmetic op=AND(invert w265, w264) -> (w301:bool)
    n189 = feedback-in #21(w301) -> ()
    n190 = call <instrlib>:"Detect Falling Edge.vi"("signal"=w265) -> ("edge detected"=w303:bool)  [unwired: 14 in]
    n191 = feedback-in #22(w303) -> ()
    n192 = xnode ("Register Read")("Data"=w265) -> ()  [unwired: 1 in, 1 out]
    n193 = Compound Arithmetic op=AND("scanEnabled", invert w265) -> (w266:bool)
    n194 = call "interpolationSummer.vi"("reset"=w341, "doStep"=w290, "upStep"="invMoveToDec") -> ("position"=w365:fxp<+,22,0>)  [unwired: 8 in]
    n195 = Compound Arithmetic op=AND(w290, w265) -> (w315:bool)
    n196 = feedback-in #23(w305) -> ()
    n197 = feedback #23() -> (w291:bool)  [unwired: 1 in]
    n198 = feedback #24() -> (w289:bool)  [unwired: 1 in]
    n199 = feedback-in #24(w290) -> ()
    n200 = Unbundle By Name("moveToPoint") -> ("x"=w367:fxp<+/-,16,1>, "y"=w368:fxp<+/-,16,1>)
    n201 = local read "singleDirectionScan"() -> (w308:bool)
    n202 = call "moveToGetPointsFromRAM2.vi"("Memory In"=refnum<k21> "moveToWave", "inputValid"=w315, "reset"=w341, "maxReached"=w272, "interpPosition"=w365, "adresses"=w343) -> ("outputValid"=w322:bool, "interpOutput"=w364:fxp<+/-,19,2>)  [unwired: 4 in]
    n203 = call "interpolationSummer.vi"("reset"=w342, "doStep"=w289, "upStep"="fastDecFactorInv") -> ("position"=w355:fxp<+,22,0>)  [unwired: 8 in]
    n204 = feedback #25() -> (w292:bool)  [unwired: 1 in]
    n205 = Compound Arithmetic op=AND(w290, w292) -> (w294:bool)
    n206 = call "slowInterpolationCounter.vi"("reset"=w291, "doStep"=w294, "upStep"="slowUpStep") -> ("fraction"=w348:fxp<+,28,0>, "index"=w337:u16)  [unwired: 7 in]
    n207 = feedback-in #26(w337) -> ()
    n208 = feedback #26() -> (w338:u16)  [unwired: 1 in]
    n209 = Increment(x=w337) -> (x+1=w363:u16)
    n210 = Not Equal?(x=w337, y=w338) -> (x != y?=w336:bool)
    n211 = Compound Arithmetic op=AND(w308, "scanEnabled", w264) -> (w307:bool)
    n212 = feedback-in #20(w307) -> ()
    n213 = Compound Arithmetic op=AND(w289, invert w265, "scanEnabled") -> (w314:bool)
    n214 = call "moveToGetPointsFromRAM2.vi"("Memory In"=refnum<k21> "fastAxisWave", "inputValid"=w314, "reset"=w342, "interpPosition"=w355, "adresses"=w285) -> ("interpOutput"=w353:fxp<+/-,19,2>)  [unwired: 5 in, 1 out]
    n215 = Less?(x=w363, y="outWaveSizeSlow") -> (x < y?=w293:bool)
    n216 = feedback-in #25(w293) -> ()
    n217 = Unbundle("fastBlanking") -> ("startFwd"=w282:u16, "endFwd"=w281:u16, "startBwd"=w276:u16, "endBwd"=w277:u16, "disableBlanking"=w279:bool)
    n218 = Unbundle(w285) -> ("index"=w275:u16)  [unwired: 1 out]
    n219 = feedback #27() -> (w378:fxp<+/-,18,2>)  [unwired: 1 in]
    n220 = feedback #28() -> (w375:fxp<+/-,18,2>)  [unwired: 1 in]
    n221 = Select(t=w337, s="singleDirectionScan", f=u16 0) -> (s? t:f=w362:u16)
    n222 = feedback #29() -> (w286:bool)  [unwired: 1 in]
    n223 = feedback-in #29(w266) -> ()
    n224 = Select(t=w363, s=w293, f=w362) -> (s? t:f=w349:u16)
    n225 = In Range and Coerce(upper limit=w281, x=w275, lower limit=w282) -> (In Range?=w284:bool)  [unwired: 1 out]
    n226 = In Range and Coerce(upper limit=w277, x=w275, lower limit=w276) -> (In Range?=w278:bool)  [unwired: 1 out]
    n227 = Bundle("index"=w337, "f"=w349) -> (w339:cluster{"index":u16, "f":u16})  [unwired: 1 in]
    n228 = Compound Arithmetic op=OR(w286, w266) -> (w267:bool)
    n229 = Compound Arithmetic op=OR(w279, w284, w278) -> (w283:bool)
    n230 = call "moveToGetPointsFromRAM2.vi"("Memory In"=refnum<k21> "slowAxisWave", "inputValid"=w314, "reset"=w336, "interpPosition"=w348, "adresses"=w339) -> ("outputValid"=w340:bool, "interpOutput"=w352:fxp<+/-,19,2>)  [unwired: 5 in]
    n231 = Compound Arithmetic op=AND(w267, w288, w283) -> (w274:bool)
    n232 = Bundle("interpOutput"=w353, "interpOutput"=w352) -> (w351:T34)  [unwired: 1 in]
    n233 = xnode ("FIFO Method Node")("Element"=w350, "Input Valid"=w274) -> ()  [unwired: 1 in, 2 out]
    n234 = xnode ("FIFO Method Node")("Element"=w350, "Input Valid"=w274) -> ()  [unwired: 1 in, 2 out]
    n235 = feedback #30() -> (w371:bool)  [unwired: 1 in]
    n236 = xnode ("High Throughput Multiply")("x"=w364, "y"=w378, "input valid"=w322, "ready for output (T)"=w371) -> ("x*y"=w377:fxp<+/-,18,2>, "output valid"=w379:bool)  [unwired: 1 out]
    n237 = feedback #31() -> (w373:bool)  [unwired: 1 in]
    n238 = xnode ("High Throughput Multiply")("x"=w364, "y"=w375, "input valid"=w322, "ready for output (T)"=w373) -> ("x*y"=w376:fxp<+/-,18,2>, "output valid"=w374:bool)  [unwired: 1 out]
    n239 = call "se_scaleOffsetRotateOutput1.vi"("inputValid"=w340, "scanSize"="scanSize", "outputMatrix"="outputMatrix", "scanOffset"="scanOffset", "input"=w351) -> ("outputValid"=w361:bool, "output"=w360:T18)  [unwired: 5 in]
    n240 = Unbundle By Name(w360) -> ("xOut"=w329:fxp<+/-,18,2>, "yOut"=w328:fxp<+/-,18,2>)
    n241 = Bundle("xOut"=w329, "yOut"=w328) -> (w327:T18)  [unwired: 1 in]
    n242 = xnode "Reinterpret Number"("x"=w329) -> ("y"=w392:fxp<+/-,18,17>)
    n243 = xnode "Reinterpret Number"("x"=w328) -> ("y"=w391:fxp<+/-,18,17>)
    n244 = call <instrlib>:"Detect Rising Edge.vi"("signal"=w361) -> ("edge detected"=w297:bool)  [unwired: 14 in]
    n245 = feedback #32() -> (w321:T35)  [unwired: 1 in]
    n246 = To Word Integer(number=w392) -> (16bit integer=w389:i16)
    n247 = To Word Integer(number=w391) -> (16bit integer=w388:i16)
    n248 = Bundle By Name(cluster=cluster{"x":i16, "y":i16} {"x"=0, "y"=0} ("Element"), "x"=w389, "y"=w388) -> (w333:cluster{"x":i16, "y":i16})
    n249 = feedback #33() -> (w311:bool)  [unwired: 1 in]
    n250 = call "stateSwitch.vi"("disable"=w311, "enable"=w272) -> ("state"=w312:bool)  [unwired: 9 in]
    n251 = feedback #34() -> (w313:cluster{"x":i16, "y":i16})  [unwired: 1 in]
    n252 = Select(t=w333, s=w297, f=w313) -> (s? t:f=w300:cluster{"x":i16, "y":i16})
    n253 = Select(t=w327, s=w297, f=w321) -> (s? t:f=w325:T35)
    n254 = feedback #35() -> (w320:T18)  [unwired: 1 in]
    "savedPoint" <- w320
    n255 = Unbundle(w320) -> ("xOut"=w323:fxp<+/-,18,2>, "yOut"=w324:fxp<+/-,18,2>)
    n256 = xnode "High Throughput Subtract"("x"=w367, "y"=w323) -> ("x-y"=w317:fxp<+/-,18,2>)
    n257 = xnode "High Throughput Subtract"("x"=w368, "y"=w324) -> ("x-y"=w316:fxp<+/-,18,2>)
    n258 = feedback-in #27(w316) -> ()
    n259 = feedback-in #28(w317) -> ()
    n260 = Unbundle(w320) -> ("xOut"=w318:fxp<+/-,18,2>, "yOut"=w319:fxp<+/-,18,2>)
    n261 = xnode ("High Throughput Add")("x"=w376, "y"=w318, "input valid"=w374) -> ("x+y"=w330:fxp<+/-,18,2>, "output valid"=w298:bool, "ready for input"=w372:bool)  [unwired: 1 in]
    n262 = xnode ("High Throughput Add")("x"=w377, "y"=w319, "input valid"=w379) -> ("x+y"=w331:fxp<+/-,18,2>, "ready for input"=w370:bool)  [unwired: 1 in, 1 out]
    n263 = feedback-in #30(w370) -> ()
    n264 = feedback-in #31(w372) -> ()
    n265 = Bundle("x+y"=w330, "x+y"=w331) -> (w326:T35)  [unwired: 1 in]
    n266 = xnode "Reinterpret Number"("x"=w330) -> ("y"=w383:fxp<+/-,18,17>)
    n267 = xnode "Reinterpret Number"("x"=w331) -> ("y"=w380:fxp<+/-,18,17>)
    n268 = feedback-in #32(w326) -> ()
    n269 = To Word Integer(number=w383) -> (16bit integer=w384:i16)
    n270 = To Word Integer(number=w380) -> (16bit integer=w382:i16)
    n271 = Compound Arithmetic op=AND(w312, w298) -> (w310:bool)
    n272 = feedback-in #33(w310) -> ()
    n273 = Bundle By Name(cluster=cluster{"x":i16, "y":i16} {"x"=0, "y"=0} ("Element"), "x"=w384, "y"=w382) -> (w332:cluster{"x":i16, "y":i16})
    n274 = feedback-in #34(w332) -> ()
    n275 = Compound Arithmetic op=OR(w297, w310) -> (w309:bool)
    n276 = Compound Arithmetic op=OR(w297, w298) -> (w299:bool)
    n277 = xnode ("FIFO Method Node")("Element"=w300, "Input Valid"=w299) -> ()  [unwired: 1 in, 2 out]
    n278 = feedback-in #35(w325, w309) -> ()
  }
  n279 = while {
    stop <- FALSE stop-if-true
    # "Output the X and Y voltages"
    n280 = xnode ("FIFO Method Node")("Timeout"=-1) -> ("Element"=w401:cluster{"x":i16, "y":i16})  [unwired: 1 in, 2 out]
    n281 = Unbundle By Name(w401) -> ("x"=w395:i16, "y"=w396:i16)
    "Y (slow)" <- w396
    "X (fast)" <- w395
    n282 = xnode "FPGA I/O Node"("Connector0/AO0"=w395) -> ()  [unwired: 1 in, 1 out]
    n283 = xnode "FPGA I/O Node"("Connector0/AO1"=w396) -> ()  [unwired: 1 in, 1 out]
    n284 = call "Tick Count2"() -> ("Tick Count(Ticks)"=w399:u32)
    n285 = feedback-in #36(w399) -> ()
    n286 = feedback #36() -> (w398:u32)  [unwired: 1 in]
    n287 = Subtract(x=w399, y=w398) -> (x-y=→"actualOutputRate":u32)
  }
  n288 = while {
    stop <- FALSE stop-if-true
    # "Replace with FIFo from scan engine"
    # "to delete too?"
    # "Retract on background correct to get non-interaction background"
    n289 = xnode ("Register Read")() -> ("Data"=w403:bool)  [unwired: 1 in, 1 out]
    n290 = Compound Arithmetic op=AND(w403, "allowPXIBGC") -> (w405:bool)
    n291 = Compound Arithmetic op=OR("resetBGC", w405) -> (w406:bool)
    n292 = case shown="True" w406 {
      frame False {
      }
      frame True {
        n293 = flat-sequence {
          frame #0 {
            n294 = xnode ("Register Write")("Data"=TRUE ("liftOff")) -> ()  [unwired: 1 in, 1 out]
          }
          frame #1 {
            n295 = disable-structure shown="FPGA_EXECUTION_MODE==FPGA_TARGET, Default" {
              frame condition #0 (active) {
                n296 = call "Wait"("Count(uSec)"="scannerTimeConstant") -> ()  [unwired: 1 out]
              }
              frame condition #1 {
              }
            }
          }
          frame #2 {
            n297 = xnode ("FIFO Method Node")("Element"=TRUE, "Timeout"=0) -> ()  [unwired: 1 in, 2 out]
          }
          frame #3 {
            n298 = call "Wait2"("Count(Ticks)"="bgcWaitTicks") -> ()  [unwired: 1 out]
          }
          frame #4 {
            n299 = xnode ("Register Write")("Data"=FALSE ("liftOff")) -> ()  [unwired: 1 in, 1 out]
            n300 = local write "resetBGC"(FALSE ("resetBGC")) -> ()
          }
        }
      }
    }
  }
  n301 = while {
    stop <- FALSE stop-if-true
    # "Approach-retract curve display on host"
    n302 = flat-sequence {
      frame #0 {
        n303 = call "Wait3"("Count(mSec)"="Count(mSec)") -> ()  [unwired: 1 out]
      }
      frame #1 {
        n304 = case shown="True" "transferInteraction" {
          frame False {
          }
          frame True {
            n305 = local read "waveLength"() -> (w419:u16)
            n306 = for {
              N: w419 -> [_]
              i -> [w424]
              n307 = xnode ("Memory Method Node")("Address"=w424) -> ("Data"=w423:cluster{"interaction":i16, "background":i16})  [unwired: 1 in, 1 out]
              n308 = Unbundle By Name(w423) -> ("interaction"=w421:i16)
              n309 = xnode ("FIFO Method Node")("Element"=w421, "Timeout"=0) -> ("Timed Out?"=w420:bool)  [unwired: 1 in, 1 out]
              n310 = case shown="True" w420 {
                frame False {
                }
                frame True {
                  n311 = local write "transferInteraction"(FALSE ("transferInteraction")) -> ()
                }
              }
            }
          }
        }
      }
      frame #2 {
        n312 = call <vilib>:"niFPGA Interrupt.vi"("Wait Until Cleared (F)"=TRUE, "IRQ Number (0)"=u8 5) -> ()  [unwired: 1 in]
      }
    }
  }
  n313 = while {
    stop <- FALSE stop-if-true
    # "Output the Z voltage"
    n314 = xnode ("FIFO Method Node")("Timeout"=-1) -> ("Element"=w429:i16)  [unwired: 1 in, 2 out]
    n315 = xnode "FPGA I/O Node"("Connector0/AO2"=w429) -> ()  [unwired: 1 in, 1 out]
  }
  n316 = node-c288(w17) -> ()
  n317 = node-c288(refnum<k21> "40 MHz Onboard Clock" ("Source Name")) -> (w14:T20)
  n318 = while {
    stop <- FALSE stop-if-true
    # "Read Vertical Deflection / Contact Mode"
    n319 = xnode "FPGA I/O Node"() -> ("Connector0/AI0"=w432)  [unwired: 1 in, 1 out]
    n320 = call "Wait5"("Count(Ticks)"="zDataRate") -> ()  [unwired: 1 out]
    n321 = xnode ("FIFO Method Node")("Element"=w432, "Timeout"=0) -> ()  [unwired: 1 in, 2 out]
  }
  n322 = timed-loop {
    timing: w14 -> [_]
    timing-out: [_] -> w13
    stop <- _ stop-if-true
    # "Slow fit calculations"
    n323 = xnode ("FIFO Method Node")("Ready for Output"=TRUE) -> ("Element"=w439:cluster{"a":i32, "b":i32}, "Output Valid"=w437:bool)  [unwired: 1 in, 1 out]
    n324 = feedback #37() -> (w446:bool)  [unwired: 1 in]
    n325 = xnode ("FIFO Method Node")("Ready for Output"=w446) -> ("Element"=w451:T23, "Output Valid"=w450:bool)  [unwired: 1 in, 1 out]
    n326 = Unbundle By Name(w439) -> ("a"=w440:i32, "b"=w441:i32)
    n327 = Subtract(x=w440, y=w441) -> (x-y=w442:i32)
    n328 = feedback-in #38(w442) -> ()
    n329 = feedback #38() -> (w438:i32)  [unwired: 1 in]
    n330 = feedback #39() -> (w444:bool)  [unwired: 1 in]
    n331 = call "linearFitCalc.vi"("ready for output (T)"=w444, "inputValid"=w450, "input"=w451) -> ("ready for input"=w447:bool, "outputValid"=w448:bool, "output"=w449:cluster{"slope":fxp<+/-,22,1>, "forward":bool})  [unwired: 6 in]
    n332 = feedback-in #37(w447) -> ()
    n333 = xnode ("FIFO Method Node")("Element"=w449, "Input Valid"=w448) -> ("Ready for Input"=w445:bool)  [unwired: 1 in, 1 out]
    n334 = feedback-in #39(w445) -> ()
    n335 = feedback-in #40(w437) -> ()
    n336 = feedback #40() -> (w436:bool)  [unwired: 1 in]
    n337 = xnode "Reinterpret Number"("x"=w438) -> ("y"=w443:fxp<+/-,32,1>)
    n338 = xnode ("FIFO Method Node")("Element"=w443, "Input Valid"=w436) -> ()  [unwired: 1 in, 2 out]
  }
  n339 = while {
    stop <- FALSE stop-if-true
    # "Host data transfer with holding averaging per pixel"
    n340 = xnode ("FIFO Method Node")("Timeout"=-1) -> ("Element"=w454:fxp<+/-,22,1>[])  [unwired: 1 in, 2 out]
    n341 = for {
      tunnel: w454 -> [w460] mode=indexing
      n342 = xnode ("FIFO Method Node")("Element"=w460, "Timeout"=0) -> ("Timed Out?"=→"hostTransferOverflow":bool)  [unwired: 1 in, 1 out]
    }
    n343 = call "Tick Count"() -> ("Tick Count(Ticks)"=w457:u32)
    n344 = feedback #41() -> (w458:u32)  [unwired: 1 in]
    n345 = feedback-in #41(w457) -> ()
    n346 = Subtract(x=w457, y=w458) -> (x-y=→"ticksPerPixel":u32)
  }
  n347 = node-c288(w15) -> ()
  n348 = while {
    stop <- FALSE stop-if-true
    # "Output the Step Motor voltages"
    n349 = xnode ("FIFO Method Node")("Timeout"=-1) -> ("Element"=w471:i8)  [unwired: 1 in, 2 out]
    n350 = xnode ("Memory Method Node")("Address"=w471) -> ("Data"=w469:bool[])  [unwired: 1 in, 1 out]
    n351 = Not(x=w469) -> (.not. x?=w468:bool[])
    n352 = Array To Cluster(array=w468) -> (cluster=w467:T36)
    n353 = Unbundle By Name(w467) -> ("[0]"=w466:bool, "[1]"=w465:bool, "[2]"=w464:bool, "[3]"=w463:bool)
    n354 = xnode "FPGA I/O Node"("Connector1/DIO0"=w466, "Connector1/DIO1"=w465, "Connector1/DIO2"=w464, "Connector1/DIO3"=w463) -> ()  [unwired: 4 in, 4 out]
  }
  n355 = node-c288(w19) -> ()
  n356 = while {
    stop <- FALSE stop-if-true
    # "Transfer background to host"
    n357 = feedback-in #42("readBackgroundAddress") -> ()
    n358 = feedback #42() -> (w478:u32)  [unwired: 1 in]
    n359 = Not Equal?(x="readBackgroundAddress", y=w478) -> (x != y?=w476:bool)
    n360 = xnode ("Register Read")() -> ("Data"=w474:bool)  [unwired: 1 in, 1 out]
    n361 = case shown="True" w476 {
      tunnel: "readBackgroundAddress" -> [_ w483]
      frame False {
      }
      frame True {
        n362 = xnode ("Memory Method Node")("Address"=w483) -> ("Data"=w482:cluster{"interaction":i16, "background":i16})  [unwired: 1 in, 1 out]
        n363 = Unbundle By Name(w482) -> ("background"=→"readBackground":i16, "interaction"=→"readInteraction":i16)
      }
    }
    n364 = call <instrlib>:"Detect Rising Edge.vi"("signal"=w474) -> ("edge detected"=w473:bool)  [unwired: 14 in]
    n365 = case shown="True" w473 {
      frame False {
      }
      frame True {
        n366 = call <vilib>:"niFPGA Interrupt.vi"("IRQ Number (0)"=u8 4) -> ()  [unwired: 2 in]
      }
    }
  }
  n367 = node-c288(w21) -> ()
  n368 = node-c288() -> (w12:T20)  [unwired: 1 in]
  n369 = timed-loop {
    timing: w12 -> [_]
    timing-out: [_] -> w11
    stop <- _ stop-if-true
    # "Deleted AuxIn"
    n370 = xnode ("Register Read")() -> ("Data"=w486:bool)  [unwired: 1 in, 1 out]
    n371 = xnode ("FIFO Method Node")("Ready for Output"=TRUE) -> ("Element"=w524:cluster{"slope":fxp<+/-,22,1>, "forward":bool}, "Output Valid"=w502:bool)  [unwired: 1 in, 1 out]
    n372 = call <instrlib>:"Detect Rising Edge.vi"("signal"=w486) -> ("edge detected"=w501:bool)  [unwired: 14 in]
    n373 = Unbundle(w524) -> ("slope"=w519:fxp<+/-,22,1>, "forward"=w506:bool)
    n374 = xnode ("FIFO Method Node")("Ready for Output"=TRUE) -> ("Output Valid"=w485:bool)  [unwired: 1 in, 2 out]
    n375 = Compound Arithmetic op=AND(w506, w502) -> (w503:bool)
    n376 = Compound Arithmetic op=AND(invert w506, w502) -> (w504:bool)
    n377 = feedback #43() -> (w491:bool)  [unwired: 1 in]
    n378 = xnode ("FIFO Method Node")("Ready for Output"=w491) -> ("Element"=w523:fxp<+/-,22,1>, "Output Valid"=w522:bool)  [unwired: 1 in, 1 out]
    n379 = Negate(x=w523) -> (-x=w489:fxp<+/-,23,2>)
    n380 = feedback #44() -> (w498:bool)  [unwired: 1 in]
    n381 = xnode ("FIFO Method Node")("Ready for Output"=w498) -> ("Element"=w521:fxp<+/-,22,1>, "Output Valid"=w520:bool)  [unwired: 1 in, 1 out]
    n382 = feedback #45() -> (w495:bool)  [unwired: 1 in]
    n383 = xnode ("FIFO Method Node")("Ready for Output"=w495) -> ("Element"=w518:fxp<+/-,22,1>, "Output Valid"=w517:bool)  [unwired: 1 in, 1 out]
    n384 = feedback #46() -> (w493:bool)  [unwired: 1 in]
    n385 = xnode ("FIFO Method Node")("Ready for Output"=w493) -> ("Element"=w516:fxp<+/-,18,1>, "Output Valid"=w515:bool)  [unwired: 1 in, 1 out]
    n386 = call "fxpAvgSCTL.vi"("reset"=w485, "clear"=w501, "inputValid"=w522, "input"=w489) -> ("outputValid"=w492:bool, "noAvg"=w508:u16, "average"=w514:fxp<+/-,22,1>, "readyForInput"=w500:bool)  [unwired: 4 in]
    n387 = feedback-in #43(w500) -> ()
    n388 = call "fxpAvgSCTL.vi"("reset"=w485, "clear"=w501, "inputValid"=w520, "input"=w521) -> ("average"=w513:fxp<+/-,22,1>, "readyForInput"=w499:bool)  [unwired: 4 in, 2 out]
    n389 = feedback-in #44(w499) -> ()
    n390 = call "fxpAvgSCTL.vi"("reset"=w485, "clear"=w501, "inputValid"=w503, "input"=w519) -> ("average"=w512:fxp<+/-,22,1>)  [unwired: 4 in, 3 out]
    n391 = call "fxpAvgSCTL.vi"("reset"=w485, "clear"=w501, "inputValid"=w517, "input"=w518) -> ("average"=w511:fxp<+/-,22,1>, "readyForInput"=w496:bool)  [unwired: 4 in, 2 out]
    n392 = feedback-in #45(w496) -> ()
    n393 = call "fxpAvgSCTL.vi"("reset"=w485, "clear"=w501, "inputValid"=w515, "input"=w516) -> ("average"=w510:fxp<+/-,22,1>, "readyForInput"=w494:bool)  [unwired: 4 in, 2 out]
    n394 = feedback-in #46(w494) -> ()
    n395 = call "fxpAvgSCTL.vi"("reset"=w485, "clear"=w501, "inputValid"=TRUE ("Output Valid"), "input"=fxp<+/-,16,1> 0.0 ("Element")) -> ("average"=w509:fxp<+/-,22,1>)  [unwired: 4 in, 3 out]
    n396 = call "fxpAvgSCTL.vi"("reset"=w485, "clear"=w501, "inputValid"=w504) -> ("average"=w505:fxp<+/-,22,1>)  [unwired: 5 in, 3 out]
    n397 = xnode "Reinterpret Number"("x"=w508) -> ("y"=w507:fxp<+,16,1>)
    n398 = Build Array(w514, w513, w512, w505, w511, w510, w509, w507) -> (w490:fxp<+/-,23,2>[])
    n399 = xnode ("FIFO Method Node")("Element"=w490, "Input Valid"=w492) -> ()  [unwired: 1 in, 2 out]
  }
  n400 = while {
    stop <- FALSE stop-if-true
    # "Pixel Synchronization"
    n401 = flat-sequence {
      frame #0 {
        n402 = xnode ("FIFO Method Node")("Timeout"=-1) -> ()  [unwired: 1 in, 3 out]
      }
      frame #1 {
        n403 = call "Tick Count3"() -> ("Tick Count(Ticks)"=w529:u32)
        n404 = feedback #47() -> (w530:u32)  [unwired: 1 in]
        n405 = feedback-in #47(w529) -> ()
        n406 = Subtract(x=w529, y=w530) -> (x-y=→"ticksPerPixel 2":u32)
      }
      frame #2 {
        n407 = call "Wait4"("Count(Ticks)"=u32 10) -> ()  [unwired: 1 out]
      }
    }
  }
  n408 = node-c288(w13) -> ()
  n409 = while {
    stop <- FALSE stop-if-true
    n410 = xnode ("FIFO Read")("Timeout"=-1) -> ("Element"=w534:i16)  [unwired: 1 in, 2 out]
    n411 = To Word Integer(number=w534) -> (16bit integer=w535:i16)
    n412 = xnode "FPGA I/O Node"("Connector0/AO7"=w535) -> ()  [unwired: 1 in, 1 out]
  }
  n413 = node-c288() -> (w2:T20)  [unwired: 1 in]
  n414 = node-c288() -> (w6:T20)  [unwired: 1 in]
  n415 = timed-loop {
    timing: w2 -> [_]
    timing-out: [_] -> w1
    stop <- _ stop-if-true
    # "Do slow move"
    n416 = case shown="True" "doSlowMove" {
      frame False {
      }
      frame True {
        n417 = xnode ("FIFO Method Node")("Element"=FALSE, "Timeout"=0) -> ()  [unwired: 1 in, 2 out]
        n418 = local write "doSlowMove"(FALSE ("doSlowMove")) -> ()
      }
    }
  }
  n419 = timed-loop {
    timing: w6 -> [_]
    timing-out: [_] -> w5
    stop <- _ stop-if-true
    # "Write adress to step motor"
    n420 = feedback #48() -> (w543:i8)  [unwired: 1 in]
    n421 = feedback-in #48("stepMot.Address(0-7)") -> ()
    n422 = Not Equal?(x="stepMot.Address(0-7)", y=w543) -> (x != y?=w545:bool)
    n423 = xnode ("FIFO Method Node")("Element"="stepMot.Address(0-7)", "Input Valid"=w545) -> ()  [unwired: 1 in, 2 out]
  }
  n424 = node-c288(w1) -> ()
  n425 = node-c288(w5) -> ()
  n426 = node-c288(w3) -> ()
  n427 = node-c288(w11) -> ()
